vi "Get Destination Directory.vi"(8 "error in":errorcluster, 11 "Build Spec in":T1) -> (0 "error out":errorcluster, 3 "Build Spec out":T1, 4 "Destination Type":string, 6 "Target Destination Directory":path)   [LabVIEW 2019, in "Project Sync Tools.lvclass"]
uses:
  Project Sync Tools.lvclass
  TypeDefs/BuildSpec Raw Parameters.ctl
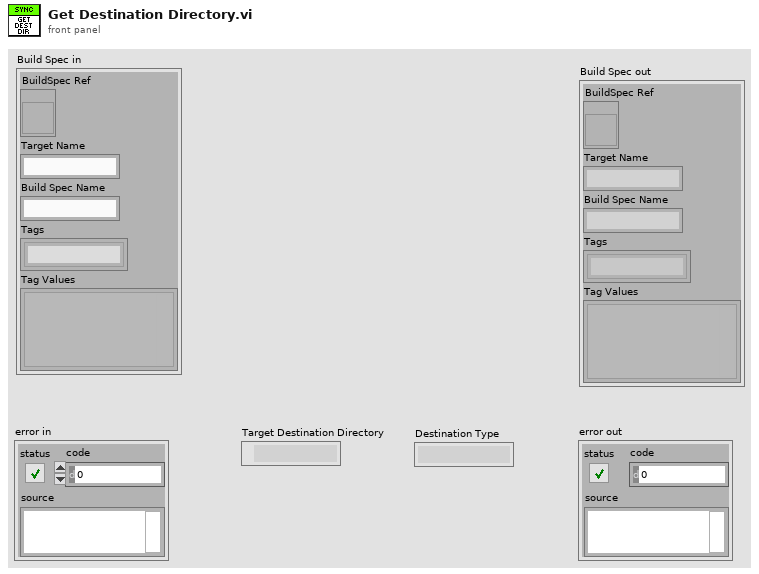
[diagram p1: front panel]
types:
  T1 = typedef "Project Sync Tools.lvclass/BuildSpec Raw Parameters.ctl" = cluster{"BuildSpec Ref":refnum<vi>, "Target Name":string, "Build Spec Name":string, "Tags":string[], "Tag Values":variant[]}
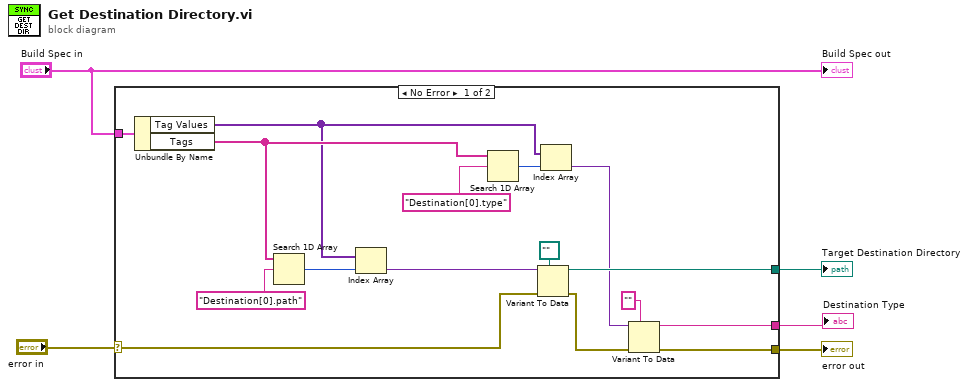
[diagram p0: block diagram]
diagram:
  n1 = case shown="No Error" "error in" {
    selector: "error in" -> [w15 w22]
    tunnel: "Build Spec in" -> [w19 _]
    tunnel: [w16 _] -> w4
    tunnel: [w7 w22] -> w3
    tunnel: [w6 _] -> w1
    frame No Error {
      n2 = Unbundle By Name(w19) -> ("Tag Values"=w12:variant[], "Tags"=w14:string[])
      n3 = Search 1D Array(1D array=w14, element="Destination[0].path") -> (index of element=w21:i32)  [unwired: 1 in]
      n4 = Index Array(array=w12, index=w21) -> (element=w18:variant)
      n5 = Search 1D Array(1D array=w14, element="Destination[0].type") -> (index of element=w11:i32)  [unwired: 1 in]
      n6 = Variant To Data(error in=w15, type=path "", Variant=w18) -> (data=w16:path, error out=w10:errorcluster)
      n7 = Index Array(array=w12, index=w11) -> (element=w9:variant)
      n8 = Variant To Data(error in=w10, type="" ("element"), Variant=w9) -> (data=w6:string, error out=w7:errorcluster)
    }
    frame Error {
    }
  }
  "Target Destination Directory" <- w4
  "error out" <- w3
  "Destination Type" <- w1
  "Build Spec out" <- "Build Spec in"
